vi "rad_Save Config.vi"(8 "error in (no error":errorcluster, 11 "State":T1 {"Targets Information"."Primary NIC"."IP Address Request Mode" items=["Static"=1, "DHCP/Link-Local"=2, "Link-Local Only"=4, "DHCP Only"=8]}) -> (0 "error out":errorcluster, 2 "Configuration File Path":path)   [LabVIEW 2020]
uses:
  TypeDefs/rad_State Data.ctl
  Targets/TypeDefs/rad_Targets Settings.ctl
  support/SubVIs/Target Information.ctl
  Targets/TypeDefs/rad_Target Network Settings.ctl
  support/Controls/Discovery Settings.ctl
  support/Controls/Discovery Method Enum.ctl
  support/Controls/Important Paths.ctl
  <vilib>/Utility/config.llb/Write Key (Boolean).vi
  rad_Globals.vi
  <vilib>/Utility/config.llb/Write Key (String).vi
  <vilib>/Utility/config.llb/Write Key (I32).vi
  <vilib>/Utility/config.llb/Write Key (Path).vi
  <vilib>/Utility/config.llb/NI_LVConfig.lvlib
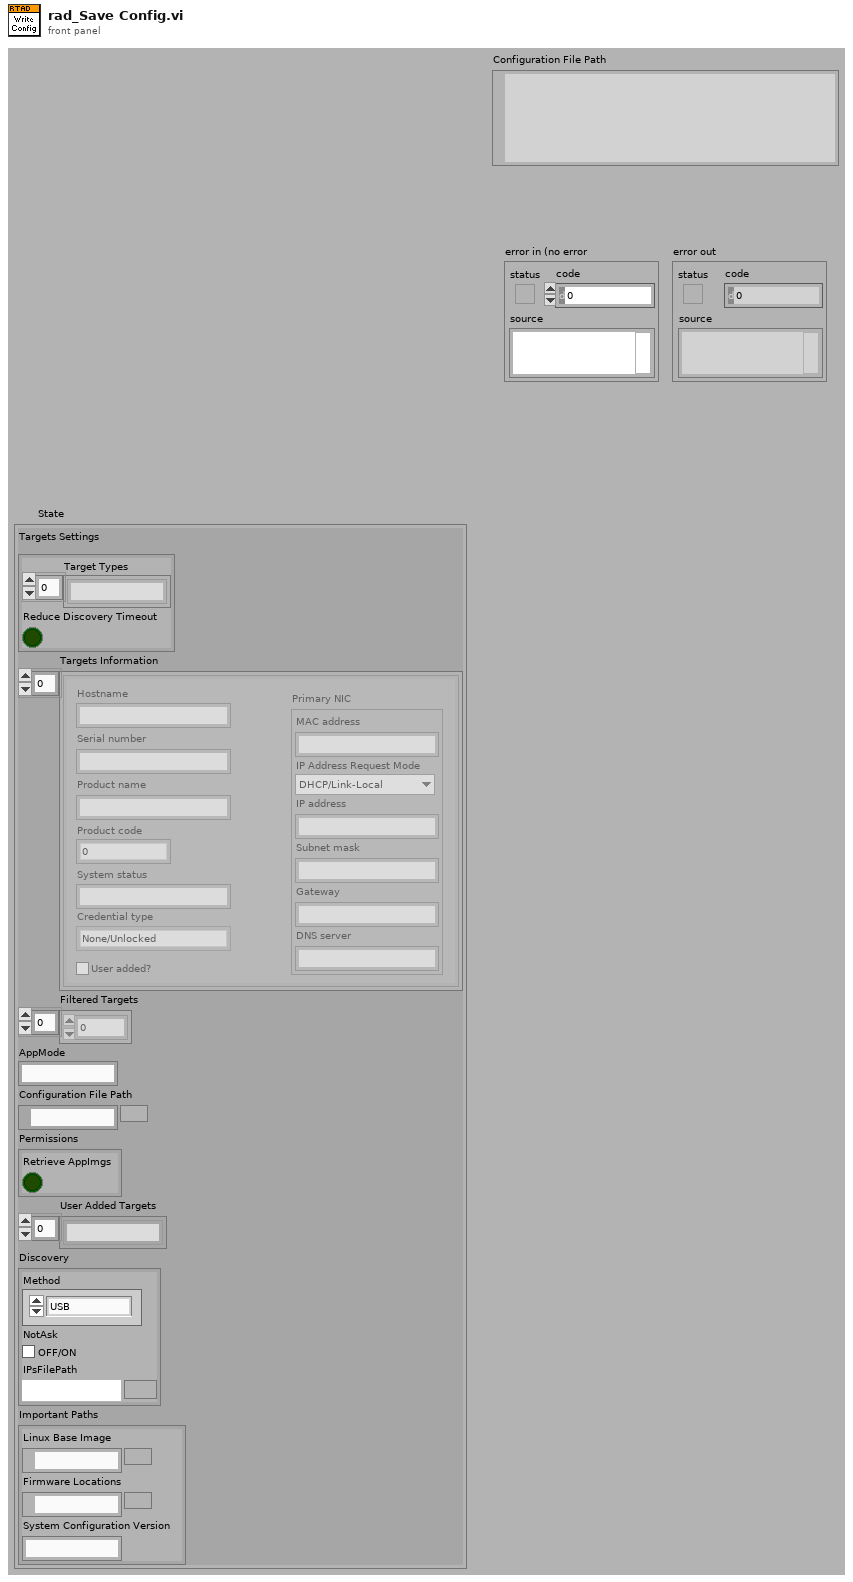
[diagram p1: front panel]
types:
  T1 = typedef "rad_State Data.ctl" = cluster{"Targets Settings":T2, "Targets Information":T3[], "Filtered Targets":i32[], "AppMode":string, "Configuration File Path":path, "Permissions":cluster{"Retrieve AppImgs":bool}, "User Added Targets":string[], "Discovery":T5, "Important Paths":T7}
  T2 = typedef "rad_Targets Settings.ctl" = cluster{"Target Types":string[], "Reduce Discovery Timeout":bool}
  T3 = typedef "Target Information.ctl" = cluster{"Hostname":string, "Serial number":string, "Product name":string, "Product code":i32, "System status":string, "Credential type":enum16{"None/Unlocked", "FTP Password", "NIAuth Credentials"}, "User added?":bool, "Primary NIC":T4}
  T4 = typedef "rad_Target Network Settings.ctl" = cluster{"MAC address":string, "IP Address Request Mode":i32, "IP address":string, "Subnet mask":string, "Gateway":string, "DNS server":string}
  T5 = typedef "Discovery Settings.ctl" = cluster{"Method":T6, "NotAsk":bool, "IPsFilePath":path}
  T6 = typedef "Discovery Method Enum.ctl" = enum32{"USB", "IPsFile", "AutoAll", "NotDiscover"}
  T7 = typedef "Important Paths.ctl" = cluster{"Linux Base Image":path, "Firmware Locations":path, "System Configuration Version":string}
  T8 = typedef "NI_LVConfig.lvlib/Config Data RefNum.ctl" = refnum<k1>
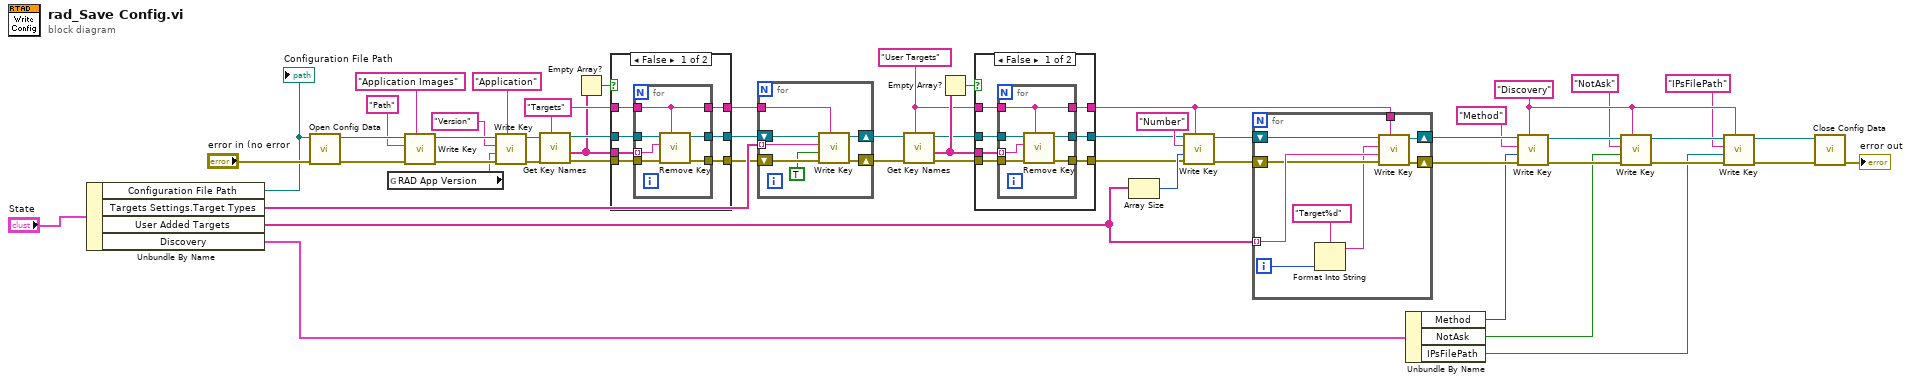
[diagram p0: block diagram]
diagram:
  w8 = "Discovery" ("section")
  w26 = "User Targets" ("section")
  w50 = "Targets" ("section")
  n1 = Unbundle By Name("State") -> ("Configuration File Path"=w16:path, "Targets Settings.Target Types"=w49:string[], "User Added Targets"=w25:string[], "Discovery"=w4:T5)
  "Configuration File Path" <- w16
  n2 = call <vilib>:"Open Config Data.vi"("error in (no error)"="error in (no error", "configuration file path"=w16) -> ("error out"=w54:errorcluster, "refnum"=w53:T8)  [unwired: 7 in, 1 out]
  n3 = global read "rad_Globals.vi" "RAD App Version"() -> (w18:string)
  n4 = call-poly <vilib>:"Write Key.vi"("section"="Application Images", "error in (no error)"=w54, "key"="Path", "refnum"=w53) -> ("error out"=w23:errorcluster, "refnum out"=w24:T8)  [unwired: 2 in, 4 out]
  n5 = call-poly <vilib>:"Write Key.vi"("section"="Application", "error in (no error)"=w23, "value"=w18, "key"="Version", "refnum"=w24) -> ("error out"=w19:errorcluster, "refnum out"=w20:T8)  [unwired: 1 in, 4 out]
  n6 = call <vilib>:"Get Key Names.vi"("section"=w50, "error in (no error)"=w19, "refnum"=w20) -> ("error out"=w51:errorcluster, "key names"=w45:string[], "refnum out"=w46:T8)  [unwired: 6 out]
  n7 = Empty Array?(array=w45) -> (empty?=w44:bool)
  n8 = case shown="False" w44 {
    tunnel: w51 -> [w62 w69]
    tunnel: w45 -> [w61 _]
    tunnel: w50 -> [w60 w71]
    tunnel: w46 -> [w59 w70]
    tunnel: [w56 w71] -> w43
    tunnel: [w58 w70] -> w42
    tunnel: [w57 w69] -> w41
    frame False {
      n9 = for {
        tunnel: w62 -> [w68]
        tunnel: w59 -> [w65]
        tunnel: w61 -> [w66] mode=indexing
        tunnel: w60 -> [w67]
        tunnel: [w67] -> w56
        tunnel: [w64] -> w57
        tunnel: [w63] -> w58
        n10 = call <vilib>:"Remove Key.vi"("section"=w67, "error in (no error)"=w68, "key"=w66, "refnum"=w65) -> ("error out"=w64:errorcluster, "refnum out"=w63:T8)  [unwired: 6 out]
      }
    }
    frame True {
    }
  }
  n11 = for {
    tunnel: w49 -> [w75] mode=indexing
    tunnel: w43 -> [w72]
    shift-right: [w74] -> w31
    shift-left: w42 -> [w78]
    shift-right: [w73] -> w30
    shift-left: w41 -> [w77]
    n12 = call-poly <vilib>:"Write Key.vi"("section"=w72, "error in (no error)"=w77, "value"=TRUE, "key"=w75, "refnum"=w78) -> ("error out"=w73:errorcluster, "refnum out"=w74:T8)  [unwired: 1 in, 4 out]
  }
  n13 = call <vilib>:"Get Key Names.vi"("section"=w26, "error in (no error)"=w30, "refnum"=w31) -> ("error out"=w32:errorcluster, "key names"=w34:string[], "refnum out"=w33:T8)  [unwired: 6 out]
  n14 = Empty Array?(array=w34) -> (empty?=w35:bool)
  n15 = case shown="False" w35 {
    tunnel: w32 -> [w85 w92]
    tunnel: w34 -> [w84 _]
    tunnel: w26 -> [w83 w94]
    tunnel: w33 -> [w82 w93]
    tunnel: [w79 w94] -> w29
    tunnel: [w81 w93] -> w28
    tunnel: [w80 w92] -> w27
    frame False {
      n16 = for {
        tunnel: w85 -> [w91]
        tunnel: w82 -> [w88]
        tunnel: w84 -> [w89] mode=indexing
        tunnel: w83 -> [w90]
        tunnel: [w90] -> w79
        tunnel: [w87] -> w80
        tunnel: [w86] -> w81
        n17 = call <vilib>:"Remove Key.vi"("section"=w90, "error in (no error)"=w91, "key"=w89, "refnum"=w88) -> ("error out"=w87:errorcluster, "refnum out"=w86:T8)  [unwired: 6 out]
      }
    }
    frame True {
    }
  }
  n18 = Array Size(array=w25) -> (size(s)=w40:i32)
  n19 = call-poly <vilib>:"Write Key.vi"("section"=w29, "error in (no error)"=w27, "value"=w40, "key"="Number", "refnum"=w28) -> ("error out"=w37:errorcluster, "refnum out"=w38:T8)  [unwired: 1 in, 4 out]
  n20 = for {
    tunnel: w25 -> [w101] mode=indexing
    tunnel: w29 -> [w102]
    shift-right: [w99] -> w36
    shift-left: w37 -> [w100]
    shift-right: [w98] -> w13
    shift-left: w38 -> [w103]
    i -> [w96]
    n21 = Format Into String(format string="Target%d", w96) -> (resulting string=w95:string)  [unwired: 2 in, 1 out]
    n22 = call-poly <vilib>:"Write Key.vi"("section"=w102, "error in (no error)"=w100, "value"=w101, "key"=w95, "refnum"=w103) -> ("error out"=w99:errorcluster, "refnum out"=w98:T8)  [unwired: 1 in, 4 out]
  }
  n23 = Unbundle By Name(w4) -> ("Method"=w3:T6, "NotAsk"=w2:bool, "IPsFilePath"=w1:path)
  n24 = call-poly <vilib>:"Write Key.vi"("section"=w8, "error in (no error)"=w36, "value"=w3, "key"="Method", "refnum"=w13) -> ("error out"=w14:errorcluster, "refnum out"=w12:T8)  [unwired: 4 in, 1 out]
  n25 = call-poly <vilib>:"Write Key.vi"("section"=w8, "error in (no error)"=w14, "value"=w2, "key"="NotAsk", "refnum"=w12) -> ("error out"=w15:errorcluster, "refnum out"=w10:T8)  [unwired: 4 in, 1 out]
  n26 = call-poly <vilib>:"Write Key.vi"("section"=w8, "error in (no error)"=w15, "value"=w1, "key"="IPsFilePath", "refnum"=w10) -> ("error out"=w11:errorcluster, "refnum out"=w9:T8)  [unwired: 4 in, 1 out]
  n27 = call <vilib>:"Close Config Data.vi"("error in (no error)"=w11, "refnum"=w9) -> ("error out"=→"error out":errorcluster)  [unwired: 1 in, 8 out]
